vi "WSVCAP SHL Host TL I2C Write.vi"(0 "C1 Data Out":u8[][](array[numeric]) format="%.0x", 5 "C2 Data Out":u8[][](array[numeric]) format="%.0x", 7 "C3 Data Out":u8[][](array[numeric]) format="%.0x", 9 "Socket Mask Set [U64]":u64[](array[numeric]) format="%012x", 11 "error in":errorcluster, 12 "Sub Address":u8=20, 13 "Log (T)":bool=TRUE) -> (15 "error out":errorcluster)   [LabVIEW 2012]
uses:
  Type Defs/WSVCAP SHL Function Enum.ctl
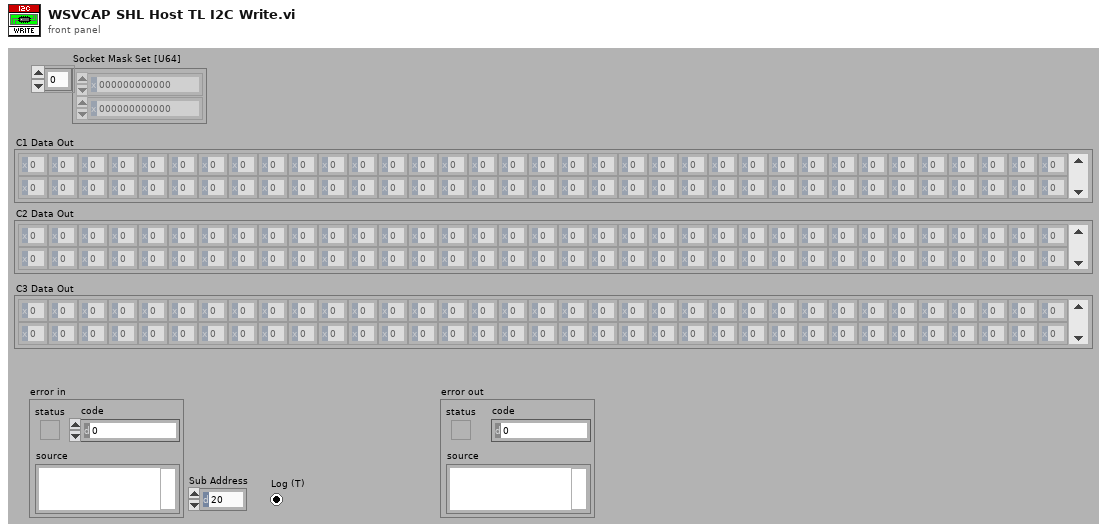
[diagram p1: front panel]
types:
  T1 = typedef "WSVCAP SHL Function Enum.ctl" = enum16{"Initialize", "Configure I2C", "Configure SPI", "Configure RFFE", "Write I2C", "Read I2C", "Write/Read SPI", "Start SPI Cycle", "Stop SPI Cycle", "Write RFFE", "Read RFFE", "Start RFFE Cycle", "Stop RFFE Cycle", "Get Status", "Close"}
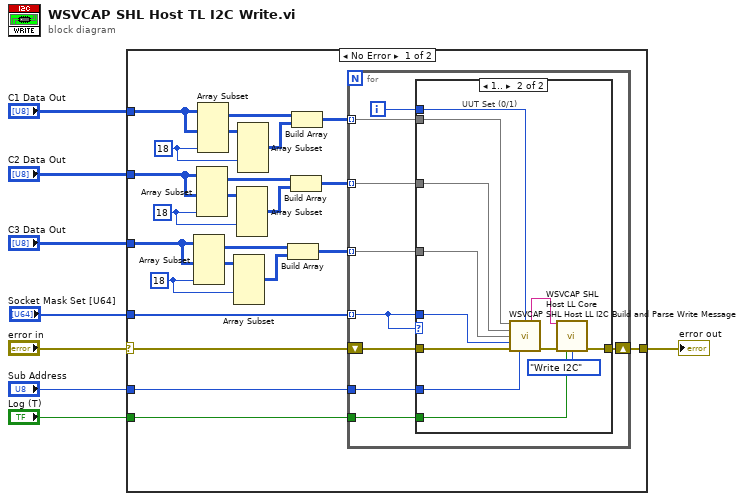
[diagram p0: block diagram]
diagram:
  n1 = case shown="No Error" "error in" {
    selector: "error in" -> [w27 w51]
    tunnel: [w28 w51] -> w8
    tunnel: "C1 Data Out" -> [w23 _]
    tunnel: "C2 Data Out" -> [w14 _]
    tunnel: "Sub Address" -> [w24 _]
    tunnel: "Socket Mask Set [U64]" -> [w26 _]
    tunnel: "Log (T)" -> [w25 _]
    tunnel: "C3 Data Out" -> [w11 _]
    frame No Error {
      w16 = 18 ("length")
      w17 = 18 ("length")
      w22 = 18 ("length")
      n2 = Array Subset(array=w11, length (col)=w16) -> (w10:u8[][])  [unwired: 3 in]
      n3 = Array Subset(array=w14, length (col)=w17) -> (w13:u8[][])  [unwired: 3 in]
      n4 = Array Subset(array=w23, length (col)=w22) -> (w21:u8[][])  [unwired: 3 in]
      n5 = Array Subset(array=w11, index (col)=w16) -> (w15:u8[][])  [unwired: 3 in]
      n6 = Array Subset(array=w14, index (col)=w17) -> (w18:u8[][])  [unwired: 3 in]
      n7 = Array Subset(array=w23, index (col)=w22) -> (w20:u8[][])  [unwired: 3 in]
      n8 = Build Array(w10, w15) -> (w9:u8[][][])
      n9 = Build Array(w13, w18) -> (w12:u8[][][])
      n10 = Build Array(w21, w20) -> (w19:u8[][][])
      n11 = for {
        tunnel: w26 -> [w29] mode=indexing
        tunnel: w25 -> [w35]
        tunnel: w19 -> [w34] mode=indexing
        tunnel: w12 -> [w33] mode=indexing
        tunnel: w24 -> [w32]
        tunnel: w9 -> [w31] mode=indexing
        shift-right: [w37] -> w28
        shift-left: w27 -> [w36]
        i -> [w30]
        n12 = case shown="1.." w29 {
          tunnel: [w38 w49] -> w37
          tunnel: w36 -> [w38 w48]
          tunnel: w29 -> [_ w45]
          tunnel: w35 -> [_ w44]
          tunnel: w34 -> [_ w43]
          tunnel: w33 -> [_ w42]
          tunnel: w32 -> [_ w41]
          tunnel: w31 -> [_ w40]
          tunnel: w30 -> [_ w39]
          frame ..0 {
          }
          frame 1.. {
            # "UUT Set (0/1)"
            n13 = call "WSVCAP SHL Host LL I2C Build and Parse Write Message.vi"("C1 Write Data In [DUT Ordered]"=w43, "UUT Set (0/1) In"=w39, "C2 Write Data [DUT Ordered]"=w42, "C3Write Data [DUT Ordered]"=w40, "Socket Mask [U64] In"=w45, "error in"=w48, "Sub Address In"=w41) -> ("Message Out"=w46:string, "error out"=w47:errorcluster)  [unwired: 1 in, 6 out]
            n14 = call "WSVCAP SHL Host LL Core.vi"("Message In"=w46, "error in"=w47, "Log (T)"=w44, "Function"=WSVCAP_SHL_Function_Enum."Write I2C") -> ("error out"=w49:errorcluster)  [unwired: 9 in, 2 out]
          }
        }
      }
    }
    frame Error {
    }
  }
  "error out" <- w8
